vi "NI-RFSG_Enable Output.vi"(8 "error in":errorcluster, 10 "Enable?":bool=TRUE, 11 "Handle In":variant) -> (0 "error out":errorcluster {"code" format="%.0x"}, 3 "Handle Out":variant)   [LabVIEW 2015]
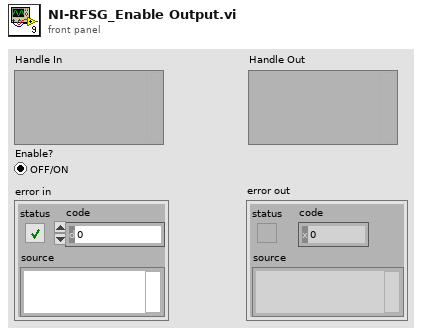
[diagram p1: front panel]
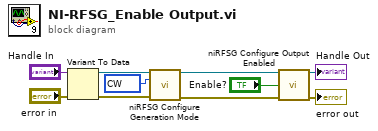
[diagram p0: block diagram]
diagram:
  w10 = 1000 items=["CW"=1000, "Arb Waveform"=1001, "Script"=1002] ("generation mode")
  n1 = Variant To Data(error in="error in", Variant="Handle In") -> (data=w6:refnum<k15>, error out=w5:errorcluster)  [unwired: 1 in]
  n2 = call <instrlib>:"niRFSG Configure Generation Mode.vi"("instrument handle"=w6, "generation mode"=w10, "error in"=w5) -> ("instrument handle out"=w8:refnum<k15>, "error out"=w7:errorcluster)  [unwired: 11 in]
  n3 = call <instrlib>:"niRFSG Configure Output Enabled.vi"("instrument handle"=w8, "output enabled"="Enable?", "error in"=w7) -> ("instrument handle out"=→"Handle Out":refnum<k15>, "error out"=→"error out":errorcluster)  [unwired: 11 in]
